vi "Deserialize (Data).vi"(8 "error in (no error)":errorcluster, 10 "Data":refnum<class "Data.lvclass">, 11 "Data in":refnum<class "Data.lvclass">) -> (0 "error out":errorcluster, 2 "Returned data out":refnum<class "Data.lvclass">, 3 "Data out":refnum<class "Data.lvclass">)   [LabVIEW 2013, in "MDSplus.lvlib" / "Data.lvclass"]
uses:
  <vilib>/MDSplus/Classes/Data_Class/Data.lvclass
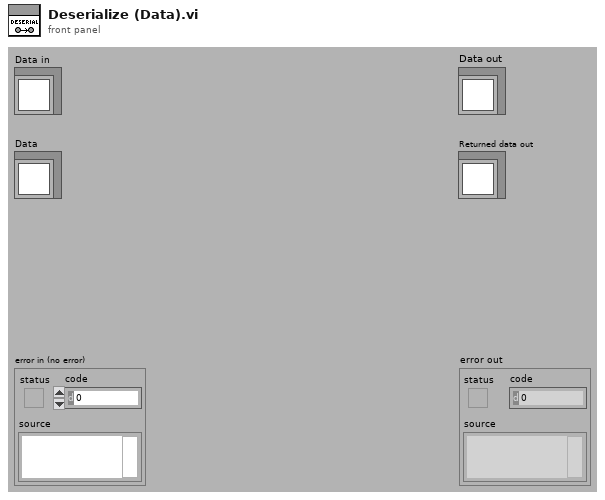
[diagram p1: front panel]
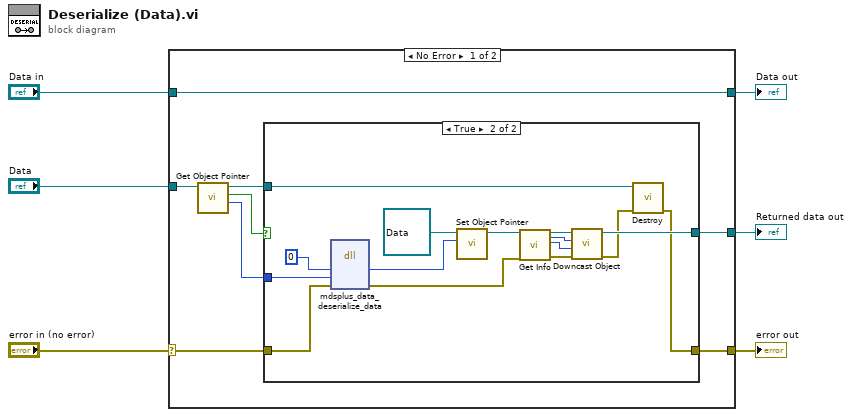
[diagram p0: block diagram]
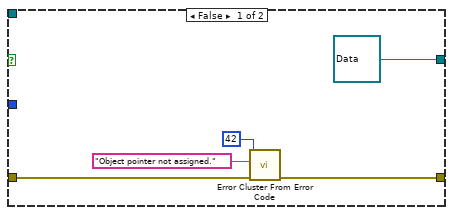
[diagram p2: hidden frame]
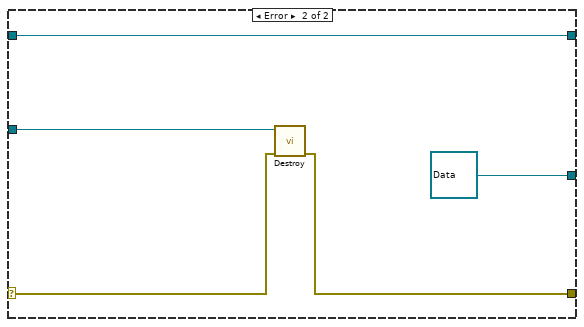
[diagram p3: hidden frame]
diagram:
  n1 = case shown="No Error" "error in (no error)" {
    selector: "error in (no error)" -> [w14 w37]
    tunnel: [w13 w36] -> w5
    tunnel: [w12 refnum<class "Data.lvclass"> refnum ("MDSplus.lvlib:Data.lvclass")] -> w4
    tunnel: "Data" -> [w11 w38]
    tunnel: [w7 w35] -> w2
    tunnel: "Data in" -> [w7 w35]
    frame No Error {
      n2 = call-dynamic "Get Object Pointer.vi"("Data in"=w11) -> ("Object Pointer"=w8:i64, "Assigned object pointer?"=w10:bool, "Data out"=w9:refnum<class "Data.lvclass">)  [unwired: 8 in]
      n3 = case shown="True" w10 {
        tunnel: w14 -> [w17 w34]
        tunnel: [w16 w20] -> w13
        tunnel: [refnum<class "Data.lvclass"> refnum ("Data out") w24] -> w12
        tunnel: w9 -> [_ w22]
        tunnel: w8 -> [_ w23]
        frame False {
          n4 = call <vilib>:"Error Cluster From Error Code.vi"("error in (no error)"=w17, "error message (\"\")"="Object pointer not assigned." ("error message (\"\")"), "error code (0)"=42) -> ("error out"=w16:errorcluster)  [unwired: 6 in]
        }
        frame True {
          n5 = dll-call lib="MDSobjectsLVShr" fn="mdsplus_data_deserialize_data"("lvDataPtrOut"=i64 0 ("lvTreeNodePtr"), "lvDataPtrIn"=w23, "error"=w34) -> ("lvDataPtrOut"=w26:i64, "error"=w25:errorcluster)  [unwired: 5 in, 2 out]
          n6 = call-dynamic "Set Object Pointer.vi"("Object Pointer"=w26, "Data in"=refnum<class "Data.lvclass"> refnum ("Data.lvclass")) -> ("Data out"=w31:refnum<class "Data.lvclass">)  [unwired: 9 in]
          n7 = call-dynamic "Get Info.vi"("Data in"=w31, "error in (no error)"=w25) -> ("Data out"=w30:refnum<class "Data.lvclass">, "Class type out"=w29:u8, "Data type out"=w28:u8, "error out"=w27:errorcluster)  [unwired: 12 in, 2 out]
          n8 = call <vilib>:"Downcast Object.vi"("error in (no error)"=w27, "Data Type"=w28, "Class Type"=w29, "Data in"=w30) -> ("error out"=w21:errorcluster, "Data out"=w24:refnum<class "Data.lvclass">)  [unwired: 6 in]
          n9 = call-dynamic "Destroy.vi"("error in (no error)"=w21, "Data in"=w22) -> ("error out"=w20:errorcluster)  [unwired: 9 in]
        }
      }
    }
    frame Error {
      n10 = call-dynamic "Destroy.vi"("error in (no error)"=w37, "Data in"=w38) -> ("error out"=w36:errorcluster)  [unwired: 9 in]
    }
  }
  "error out" <- w5
  "Returned data out" <- w4
  "Data out" <- w2
